vi "read test param.vi"(8 "error in (no error)":errorcluster, 10 "File Path":path, 11 "EVI 79 in":refnum<class "EVI 79.lvclass">) -> (0 "error out":errorcluster, 3 "EVI 79 out":refnum<class "EVI 79.lvclass">)   [LabVIEW 2025, in "EVI 79.lvclass"]
uses:
  EVI 79.lvclass
  EVI 79.lvclass/EVI 79.ctl
  e6b43afd-9f1b-4e40-9abe-1c3b415931ca.vi
  <vilib>/JDP Science/JSONtext/JSON text to Variant.vi
  <vilib>/JDP Science/JSONtext/LVClass Serializer/JSONtext LVClass Serializer.lvclass
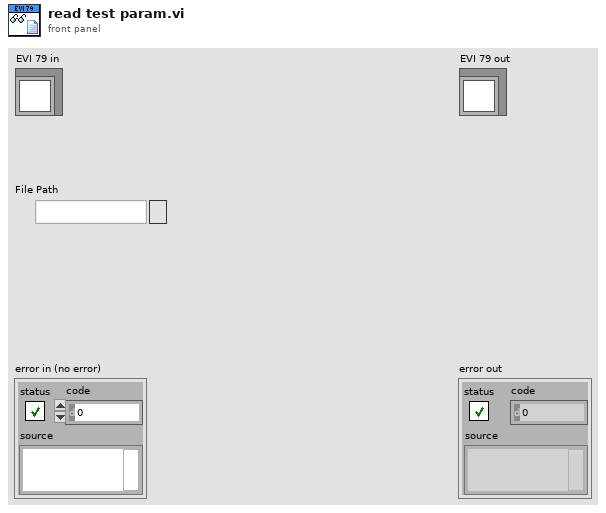
[diagram p1: front panel]
types:
  T1 = enum16{"open", "replace", "create", "open or create", "replace or create", "replace or create with confirmation"}
  T2 = cluster{"Electrical_Properties":cluster{"V_max":dbl, "I_max":dbl}, "Wear_in":cluster{"V":dbl, "I":dbl, "Cycles":dbl, "On_Time_ms":dbl, "Off_Time_ms":dbl}}
  T3 = cluster{"V":dbl, "I":dbl, "Cycles":dbl, "On_Time_ms":dbl, "Off_Time_ms":dbl}
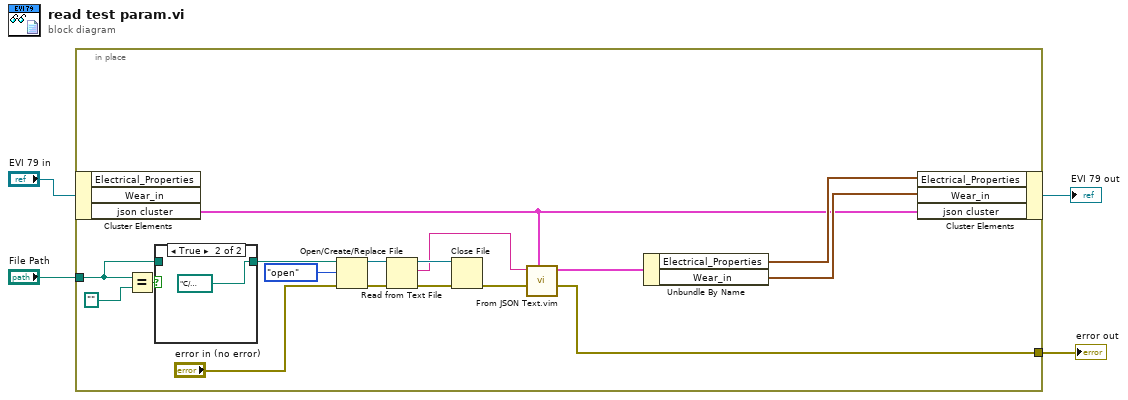
[diagram p0: block diagram]
diagram:
  n1 = in-place {
    in-place-border: "File Path" -> [w19]
    in-place-border: [w5] -> w1
    n2 = in-place-cluster #1("EVI 79 in") -> ("json cluster"=w6:T2)  [unwired: 2 out]
    n3 = Equal?(x=w19, y=path "") -> (x = y?=w20:bool)
    n4 = case shown="True" w20 {
      tunnel: [w22 path "C:/Users/Public/Documents/atp-station/programs/EVI-79-param.json" ("File Path")] -> w18
      tunnel: w19 -> [w22 _]
      frame False {
      }
      frame True {
      }
    }
    n5 = Open/Create/Replace File(file path (use dialog)=w18, error in="error in (no error)", operation (0:open)=T1."open") -> (refnum out=w15:refnum<file>, error out=w14:errorcluster)  [unwired: 3 in, 1 out]
    n6 = Read from Text File(file (use dialog)=w15, error in=w14) -> (refnum out=w12:refnum<file>, text=w11:string, error out=w13:errorcluster)  [unwired: 2 in, 1 out]
    n7 = Close File(refnum=w12, error in=w13) -> (error out=w10:errorcluster)  [unwired: 1 out]
    n8 = call "From JSON Text.vim"("Data Type and Default Value"=w6, "error in (no error)"=w10, "JSON"=w11) -> ("error out"=w5:errorcluster, "Data out"=w9:T2)  [unwired: 7 in]
    n9 = Unbundle By Name(w9) -> ("Electrical_Properties"=w8:cluster{"V_max":dbl, "I_max":dbl}, "Wear_in"=w7:T3)
    n10 = in-place-cluster #1("Electrical_Properties"=w8, "Wear_in"=w7, "json cluster"=w6) -> (→"EVI 79 out":refnum<class "EVI 79.lvclass">)
  }
  "error out" <- w1
